vi "Main.vi"() -> ()   [LabVIEW 2015]
uses:
  System.Windows.Forms
panel:
  out "Stop?":bool
  in  "Browser":refnum<k24>(container)
  in  "Search":bool
  out "String":string
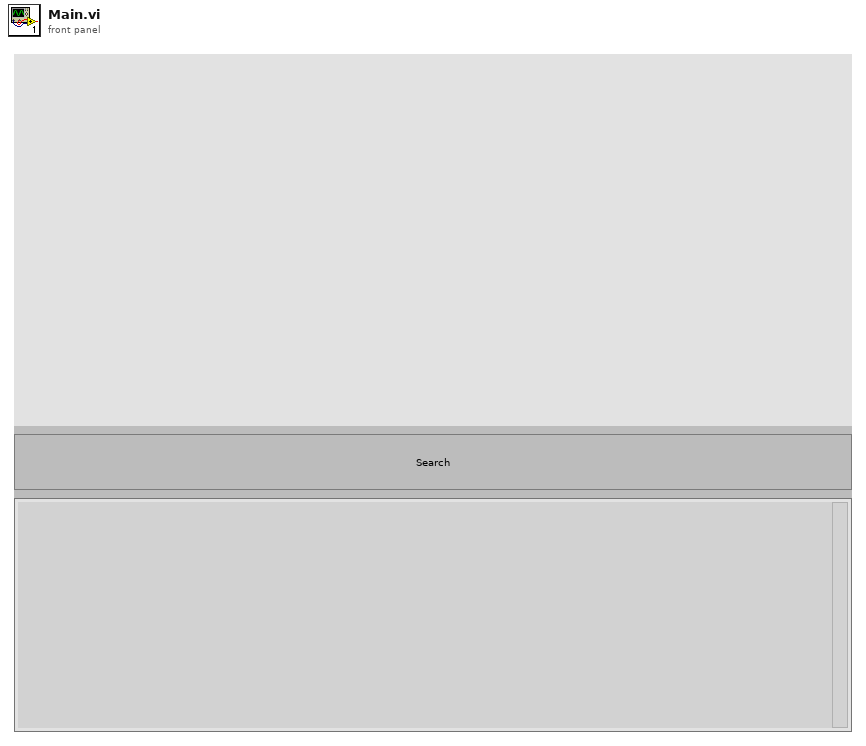
[diagram p1: front panel]
types:
  T1 = enum32{"invalid app kind", "Development System", "Run Time System", "Student Edition", "Embedded LabVIEW", "Evaluation", "Custom"}
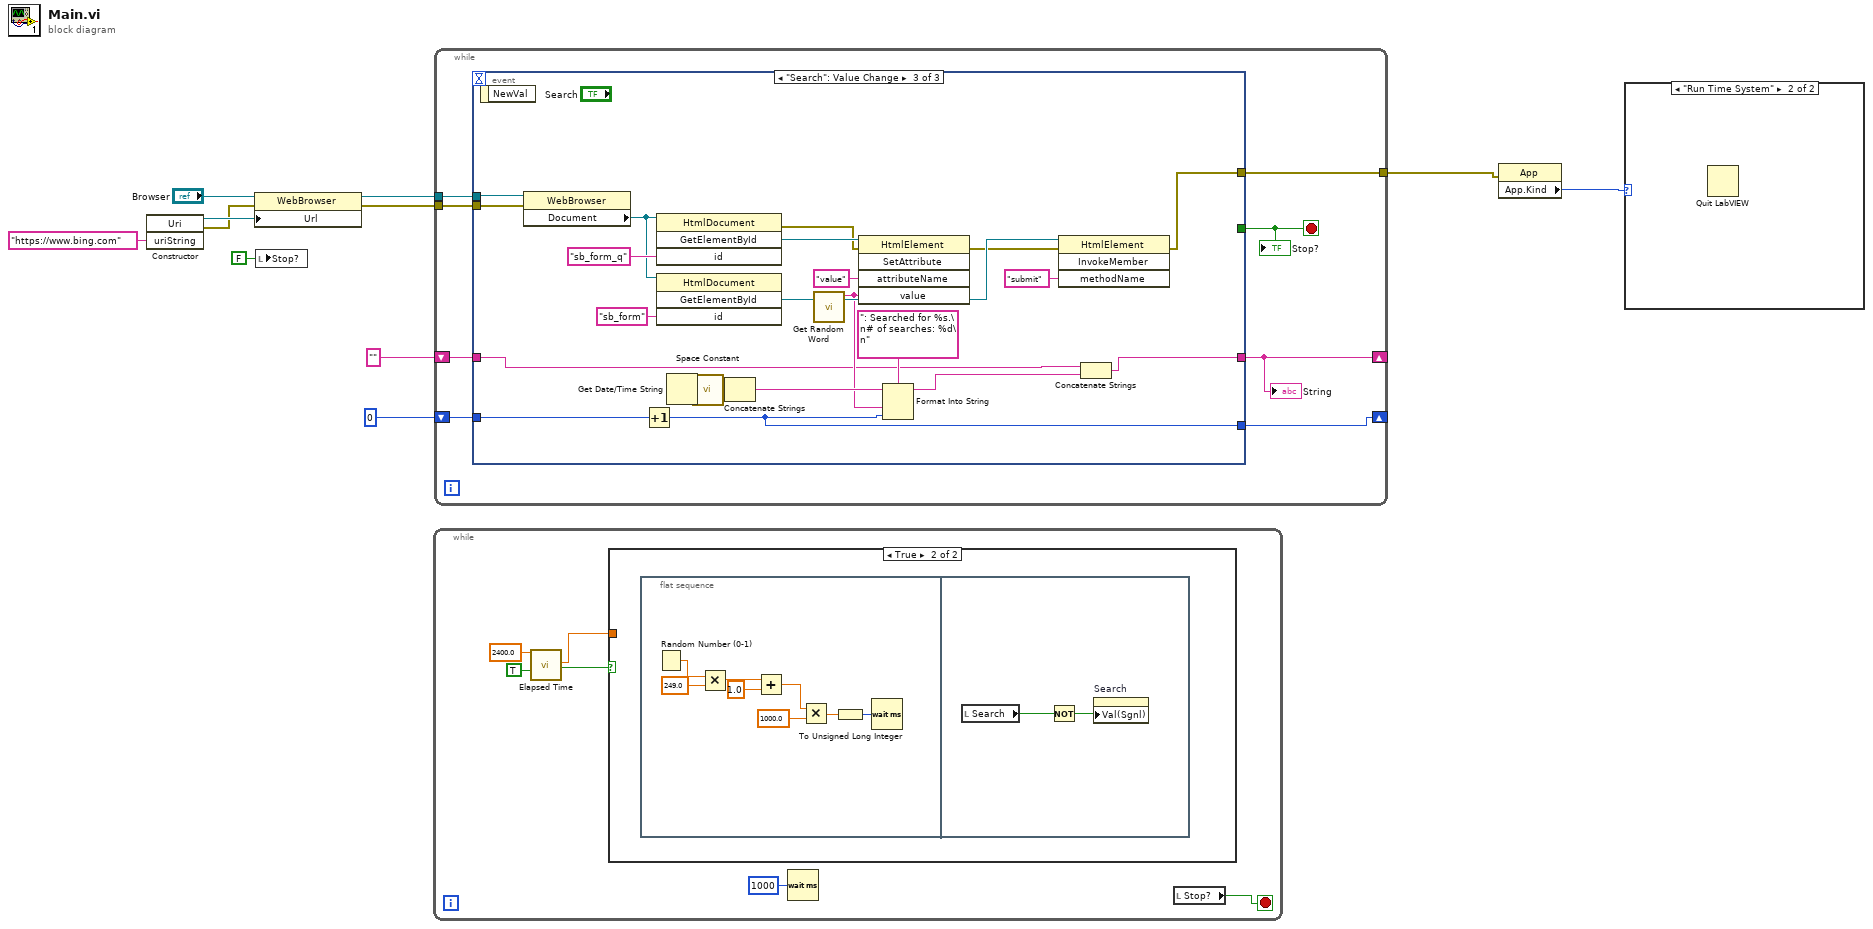
[diagram p0: block diagram]
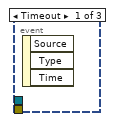
[diagram p4: hidden frame]
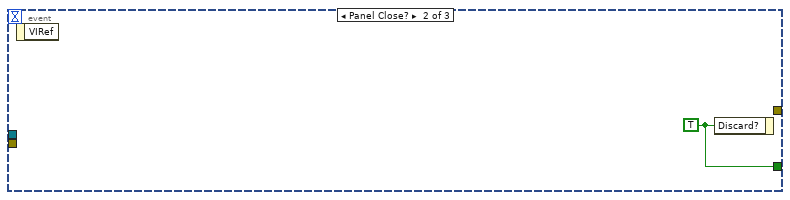
[diagram p5: hidden frame]
diagram:
  n1 = constructor class="Uri"("uriString"="https://www.bing.com") -> (reference out=w9:refnum<k24>, error out=w7:errorcluster)  [unwired: 3 in, 2 out]
  n2 = property class="WebBrowser"(reference="Browser", error in=w7, "Url"=w9) -> (reference out=w6:refnum<k24>, error out=w8:errorcluster)
  n3 = local write "Stop?"(FALSE ("Stop?")) -> ()
  n4 = while {
    stop <- w14 stop-if-true
    n5 = call "Elapsed Time"("Time Target (s)"=2400.0, "Auto Reset"=TRUE) -> ("Elapsed Time (s)"=w13:dbl, "Time has Elapsed"=w15:bool)  [unwired: 10 in, 6 out]
    n6 = case shown="True" w15 {
      tunnel: w13 -> [_ _]
      frame False {
      }
      frame True {
        n7 = flat-sequence {
          frame #0 {
            n8 = Random Number (0-1)() -> (number: 0 to 1=w25:dbl)
            n9 = Multiply(x=w25, y=249.0) -> (x*y=w23:dbl)
            n10 = Add(x=w23, y=1.0) -> (x+y=w21:dbl)
            n11 = Multiply(x=w21, y=1000.0) -> (x*y=w19:dbl)
            n12 = To Unsigned Long Integer(number=w19) -> (unsigned 32bit integer=w18:u32)
            n13 = Wait (ms)(milliseconds to wait=w18) -> ()  [unwired: 1 out]
          }
          frame #1 {
            n14 = local read "Search"() -> (w27:bool)
            n15 = Not(x=w27) -> (.not. x?=w26:bool)
            n16 = property on="Search" class="Bool (strict)"("Val(Sgnl)"=w26) -> ()  [unwired: 2 in, 2 out]
          }
        }
      }
    }
    n17 = Wait (ms)(milliseconds to wait=u32 1000) -> ()  [unwired: 1 out]
    n18 = local read "Stop?"() -> (w14:bool)
  }
  n19 = while {
    tunnel: w8 -> [w35]
    tunnel: w6 -> [w33]
    shift-right: [w29] -> _
    shift-left: "" -> [w32]
    shift-right: [w30] -> _
    shift-left: 0 -> [w31]
    tunnel: [w28] -> w2
    stop <- w34 stop-if-true
    n20 = event shown="[2] \"Search\": Value Change" {
      selector: _ -> [_ _ _]
      dyn-events: _ -> [_ _ _]
      timeout: _ -> [_ _ _]
      tunnel: w35 -> [_ _ w54]
      tunnel: [_ w36 _] -> w34
      tunnel: w33 -> [_ _ w55]
      tunnel: w32 -> [_ _ w40]
      tunnel: w31 -> [_ _ w42]
      tunnel: [_ _ w41] -> w30
      tunnel: [_ _ w38] -> w29
      tunnel: [_ _ w37] -> w28
      event Timeout {
        n21 = event-data() -> ()  [unwired: 1 in, 3 out]
      }
      event Panel Close? {
        w36 = TRUE ("Discard?")
        n22 = event-data() -> ()  [unwired: 1 in, 1 out]
        n23 = event-data("Discard?"=w36) -> ()  [unwired: 1 in, 1 out]
      }
      event "Search": Value Change {
        n24 = event-data() -> ()  [unwired: 1 in, 1 out]
        n25 = property class="WebBrowser"(reference=w55, error in=w54) -> ("Document"=w53:refnum<k24>)  [unwired: 2 out]
        n26 = Increment(x=w42) -> (x+1=w41:i32)
        n27 = invoke class="HtmlDocument" method="GetElementById"(reference=w53, "id"="sb_form_q") -> (error out=w51:errorcluster, "GetElementById"=w58:refnum<k24>)  [unwired: 2 in, 2 out]
        n28 = invoke class="HtmlDocument" method="GetElementById"(reference=w53, "id"="sb_form") -> ("GetElementById"=w50:refnum<k24>)  [unwired: 2 in, 3 out]
        n29 = Get Date/Time String() -> (date string=w47:string, time string=w48:string)  [unwired: 3 in]
        n30 = call <vilib>:"Space Constant.vi"() -> ("String"=w46:string)
        n31 = Concatenate Strings(w47, w46, w48) -> (w45:string)
        n32 = call "Get Random Word.vi"() -> ("element"=w43:string)  [unwired: 11 in]
        n33 = invoke class="HtmlElement" method="SetAttribute"(reference=w58, error in=w51, "attributeName"="value", "value"=w43) -> (error out=w49:errorcluster)  [unwired: 1 in, 4 out]
        n34 = Format Into String(format string=": Searched for %s.\n# of searches: %d\n", initial string=w45, w43, w41) -> (resulting string=w39:string)  [unwired: 1 in, 1 out]
        n35 = invoke class="HtmlElement" method="InvokeMember"(reference=w50, error in=w49, "methodName"="submit" ("eventName")) -> (error out=w37:errorcluster)  [unwired: 1 in, 3 out]
        n36 = Concatenate Strings(w40, w39) -> (w38:string)
      }
    }
    "Stop?" <- w34
    "String" <- w29
  }
  n37 = property class="App"(error in=w2) -> ("App.Kind"=w1:T1)  [unwired: 1 in, 2 out]
  n38 = case shown="\"Run Time System\"" w1 {
    frame "invalid app kind", Default {
    }
    frame "Run Time System" {
      n39 = Quit LabVIEW() -> ()  [unwired: 1 in]
    }
  }
